vi "Set Langauge (by VI).vi"(8 "error in":errorcluster, 9 "Target Language":string, 10 "VI Ref":refnum<vi>) -> (0 "error out":errorcluster)   [LabVIEW 2019]
doc: "Translates a single VI without adding it to the local registry.\n\nTarget Language: Optional input. Leave blank to use the default language."
uses:
  SubVIs/Localization FGV Action -- Enum.ctl
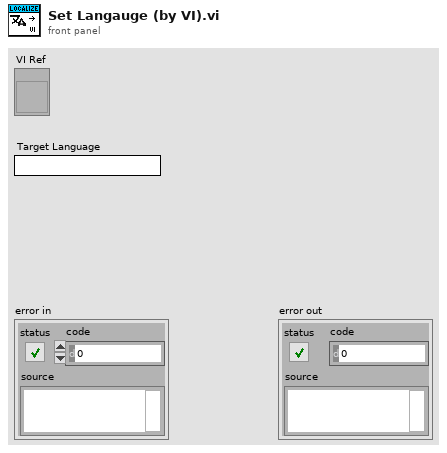
[diagram p1: front panel]
types:
  T1 = typedef "Localization FGV Action -- Enum.ctl" = enum16{"Read Dictionary", "Translate VIs", "Register VI", "Get Languages", "Translate Phrase", "Translate VI", "Unregister"}
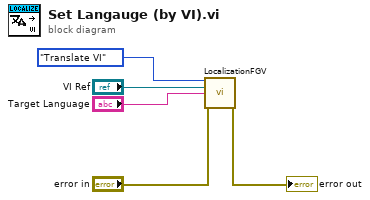
[diagram p0: block diagram]
diagram:
  n1 = call "LocalizationFGV.vi"("Action"=Localization_FGV_Action_--_Enum."Translate VI", "VI in"="VI Ref", "Target Language"="Target Language", "error in"="error in") -> ("error out"=→"error out":errorcluster)  [unwired: 7 in, 4 out]
